vi "叶绿素a_设置用户校准参数.vi"(8 "error in (no error)":errorcluster caption="错误输入（无错误）", 10 "用户校准参数":cluster{"K":sgl, "B":sgl}, 11 "MB session in":refnum<class "MB_Master.lvclass">) -> (0 "error out":errorcluster caption="错误输出", 3 "MB session out":refnum<class "MB_Master.lvclass">)   [LabVIEW 2016, in "斯坦道多参数.lvlib"]
uses:
  <vilib>/Plasmionique/MB Master/MB Master.lvlib
  <vilib>/Plasmionique/MB Master/MB_Master/MB_Master.lvclass
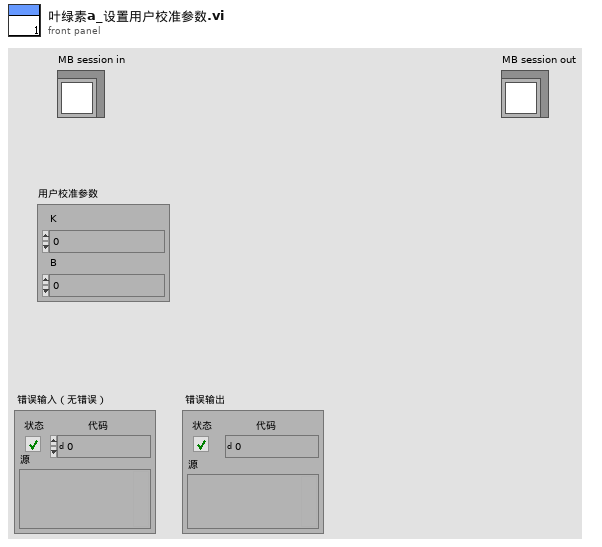
[diagram p1: front panel]
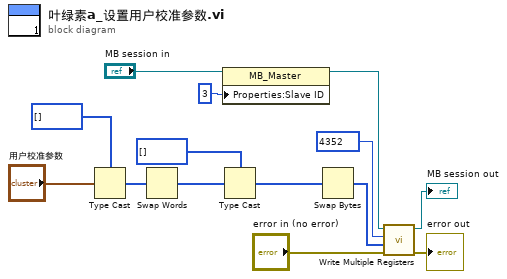
[diagram p0: block diagram]
diagram:
  n1 = Type Cast(type=u32[] [] ("数组 2"), x="用户校准参数") -> (*(type *) &x=w3:u32[])
  n2 = Swap Words(1:w3) -> (0:w8:u32[])
  n3 = property class="MB_Master"(reference="MB session in", "Properties:Slave ID"=u8 3 ("Slave ID")) -> (reference out=w11:refnum<class "MB_Master.lvclass">)  [unwired: 1 in, 1 out]
  n4 = Type Cast(type=u16[] [] ("数组 2"), x=w8) -> (*(type *) &x=w7:u16[])
  n5 = Swap Bytes(anything=w7) -> (byte swapped=w5:u16[])
  n6 = call <vilib>:"Write Multiple Registers.vi"("error in (no error)"="error in (no error)", "values"=w5, "starting address"=u16 4352, "MB session in"=w11) -> ("error out"=→"error out":errorcluster, "MB session out"=→"MB session out":refnum<class "MB_Master.lvclass">)  [unwired: 6 in]
